vi "Set control states.vi"(0 "VI Refnum":refnum<vi>, 2 "Control State(Enable)":T1(ring), 5 "error in (no error)":errorcluster, 8 "Control Names to exlude":string[](array[string])=["error in (no error)", "error out", "Debug Abort"]) -> (19 "error out":errorcluster)   [LabVIEW 2018]
doc: "Determines what controls the user would like grayed out or disabled. Once this has been determined it then disables or exludes those controls."
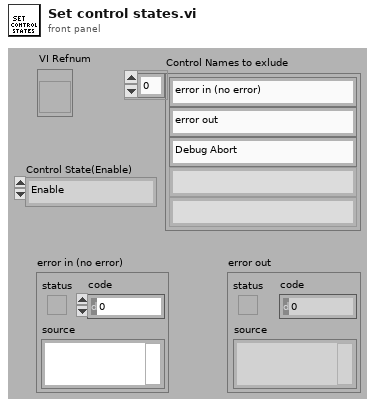
[diagram p1: front panel]
types:
  T1 = enum8{"Enable", "Disabled", "Disabled and Grayed"}
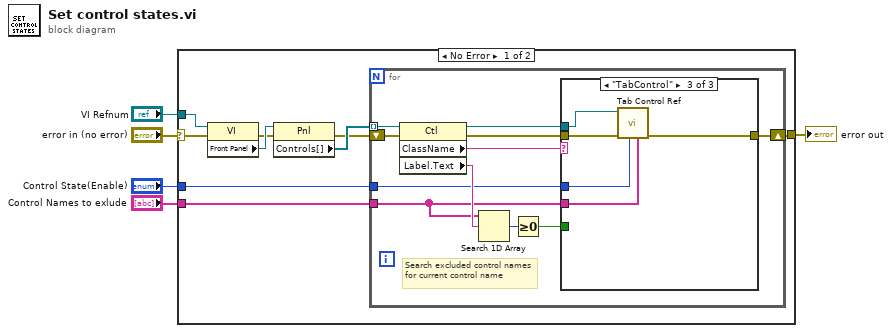
[diagram p0: block diagram]
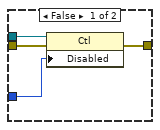
[diagram p3: hidden frame]
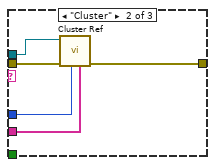
[diagram p4: hidden frame]
diagram:
  n1 = case shown="No Error" "error in (no error)" {
    selector: "error in (no error)" -> [w8 w46]
    tunnel: [w12 w46] -> w4
    tunnel: "VI Refnum" -> [w14 _]
    tunnel: "Control Names to exlude" -> [w10 _]
    tunnel: "Control State(Enable)" -> [w9 _]
    frame No Error {
      n2 = property class="VI"(reference=w14, error in=w8) -> (error out=w7:errorcluster, "Front Panel"=w13:refnum<vi>)  [unwired: 1 out]
      n3 = property class="Pnl"(reference=w13, error in=w7) -> (error out=w6:errorcluster, "Controls[]"=w11:refnum<vi>[])  [unwired: 1 out]
      n4 = for {
        shift-right: [w18] -> w12
        shift-left: w6 -> [w25]
        tunnel: w11 -> [w23] mode=indexing
        tunnel: w10 -> [w16]
        tunnel: w9 -> [w17]
        # "Search excluded control names for current control name"
        n5 = property class="Ctl"(reference=w23, error in=w25) -> (reference out=w19:refnum<vi>, error out=w20:errorcluster, "ClassName"=w21:string, "Label.Text"=w22:string)
        n6 = Search 1D Array(1D array=w16, element=w22) -> (index of element=w24:i32)  [unwired: 1 out]
        n7 = Greater Or Equal To 0?(x=w24) -> (x >= 0?=w15:bool)
        n8 = case shown="\"TabControl\"" w21 {
          tunnel: w20 -> [w30 w40 w45]
          tunnel: w19 -> [w29 w39 w44]
          tunnel: [w28 w38 w43] -> w18
          tunnel: w17 -> [w27 w37 w42]
          tunnel: w16 -> [_ w36 w41]
          tunnel: w15 -> [w26 _ _]
          frame Default {
            n9 = case shown="True" w26 {
              tunnel: w30 -> [w34 w35]
              tunnel: w29 -> [w33 _]
              tunnel: [w32 w35] -> w28
              tunnel: w27 -> [w31 _]
              frame False {
                n10 = property class="Ctl"(reference=w33, error in=w34, "Disabled"=w31) -> (error out=w32:errorcluster)  [unwired: 1 out]
              }
              frame True {
              }
            }
          }
          frame "Cluster" {
            n11 = call "Cluster Ref.vi"("Control Names to exlude"=w36, "Control State(Enable)"=w37, "error in"=w40, "Cluster Reference"=w39) -> ("error out"=w38:errorcluster)  [unwired: 7 in]
          }
          frame "TabControl" {
            n12 = call "Tab Control Ref.vi"("Control Names to exlude"=w41, "Control State(Enable)"=w42, "error in"=w45, "TabControl Reference"=w44) -> ("error out"=w43:errorcluster)  [unwired: 7 in]
          }
        }
      }
    }
    frame Error {
    }
  }
  "error out" <- w4
